vi "Read Stage Homed.vi"(8 "error in (no error)":errorcluster, 11 "Sync 2-Axis Stage Controller in":refnum<class "Sync 2-Axis Stage Controller.lvclass">) -> (0 "error out":errorcluster, 1 "Y-Axis Homed":bool, 2 "X-Axis Homed":bool, 3 "Sync 2-Axis Stage Controller out":refnum<class "Sync 2-Axis Stage Controller.lvclass">)   [LabVIEW 2022 SP3, in "Sync 2-Axis Stage Controller.lvclass"]
uses:
  Sync 2-Axis Stage Controller.lvclass
  Sync 2-Axis Stage Controller.lvclass/Sync 2-Axis Stage Controller.ctl
  Home State.ctl
  Axis Objects/iMotion Controller/iMotion Controller.lvclass
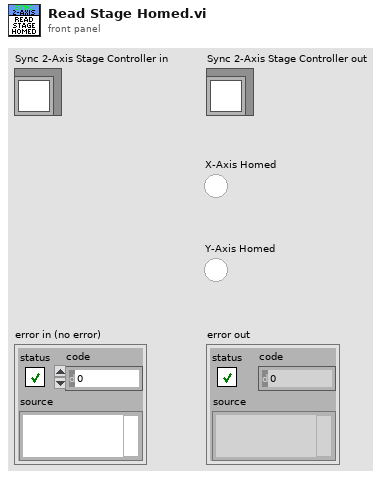
[diagram p1: front panel]
types:
  T1 = typedef "Sync 2-Axis Stage Controller.lvclass/Home State.ctl" = enum16{"Idle", "Homing 1st Axis", "Homing 2nd Axis"}
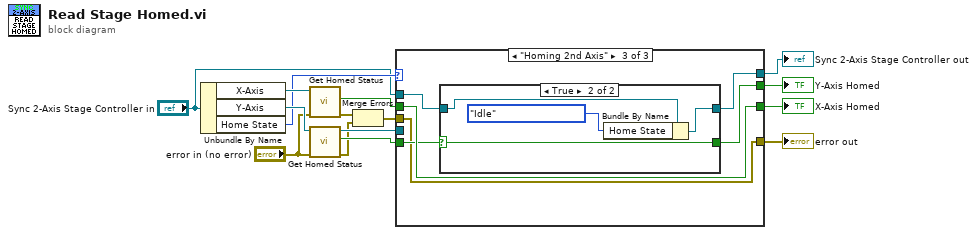
[diagram p0: block diagram]
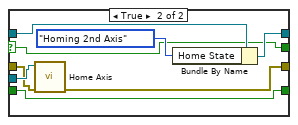
[diagram p4: hidden frame]
diagram:
  n1 = Unbundle By Name("Sync 2-Axis Stage Controller in") -> ("X-Axis"=w15:refnum<class "iMotion Controller.lvclass">, "Y-Axis"=w14:refnum<class "iMotion Controller.lvclass">, "Home State"=w13:T1)
  n2 = call-dynamic "Get Homed Status.vi"("error in (no error)"="error in (no error)", "iMotion Controller in"=w15) -> ("error out"=w2:errorcluster, "Homed"=w11:bool)  [unwired: 7 in, 1 out]
  n3 = call-dynamic "Get Homed Status.vi"("error in (no error)"="error in (no error)", "iMotion Controller in"=w14) -> ("error out"=w7:errorcluster, "Homed"=w12:bool, "iMotion Controller out"=w8:refnum<class "iMotion Controller.lvclass">)  [unwired: 7 in]
  n4 = Merge Errors(w2, w7) -> (w3:errorcluster)
  n5 = case shown="\"Homing 2nd Axis\"" w13 {
    tunnel: w12 -> [w18 w22 w45]
    tunnel: w11 -> [w19 w28 w46]
    tunnel: [w19 w23 w46] -> w10
    tunnel: [w18 w21 w44] -> w9
    tunnel: w8 -> [_ w27 _]
    tunnel: w3 -> [w16 w26 w41]
    tunnel: "Sync 2-Axis Stage Controller in" -> [w17 w25 w43]
    tunnel: [w17 w24 w42] -> w5
    tunnel: [w16 w20 w41] -> w1
    frame "Idle" {
    }
    frame "Homing 1st Axis" {
      n6 = case shown="False" w28 {
        selector: w28 -> [w31 w35]
        tunnel: w27 -> [_ w40]
        tunnel: w26 -> [w29 w39]
        tunnel: w25 -> [w32 w38]
        tunnel: [w32 w37] -> w24
        tunnel: [w31 w35] -> w23
        tunnel: w22 -> [w30 w34]
        tunnel: [w30 w34] -> w21
        tunnel: [w29 w33] -> w20
        frame False {
        }
        frame True {
          n7 = call-dynamic "Home Axis.vi"("error in (no error)"=w39, "iMotion Controller in"=w40) -> ("error out"=w33:errorcluster)  [unwired: 8 in, 1 out]
          n8 = Bundle By Name(cluster=w38, "Home State"=Home_State."Homing 2nd Axis") -> (w37:refnum<class "Sync 2-Axis Stage Controller.lvclass">)
        }
      }
    }
    frame "Homing 2nd Axis" {
      n9 = case shown="True" w45 {
        selector: w45 -> [w47 w52]
        tunnel: [w47 w52] -> w44
        tunnel: w43 -> [w48 w51]
        tunnel: [w48 w49] -> w42
        frame False {
        }
        frame True {
          n10 = Bundle By Name(cluster=w51, "Home State"=Home_State."Idle") -> (w49:refnum<class "Sync 2-Axis Stage Controller.lvclass">)
        }
      }
    }
  }
  "error out" <- w1
  "Sync 2-Axis Stage Controller out" <- w5
  "Y-Axis Homed" <- w9
  "X-Axis Homed" <- w10
